vi "Create Channel and Node Pair.vi"(8 "Port ID":string, 9 "Node ID":string, 10 "name":string, 11 "Instance ID":string) -> (3 "Channel to Port Pair":T1)   [LabVIEW 2014, in "GraphViz Mapping Visualizer.lvlib"]
uses:
  GraphViz Mapping Visualizer.lvlib
  Channel to Port Pair.ctl
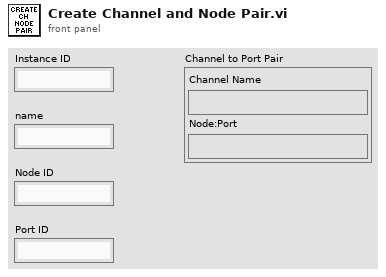
[diagram p1: front panel]
types:
  T1 = typedef "GraphViz Mapping Visualizer.lvlib/Channel to Port Pair.ctl" = cluster{"Channel Name":string, "Node:Port":string}
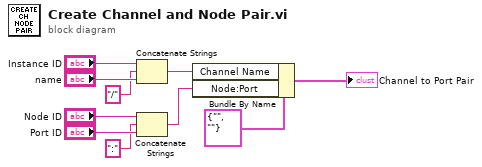
[diagram p0: block diagram]
diagram:
  n1 = Concatenate Strings("Instance ID", "/", "name") -> (w6:string)
  n2 = Concatenate Strings("Node ID", ":" ("string"), "Port ID") -> (w4:string)
  n3 = Bundle By Name(cluster=T1 {"Channel Name"="", "Node:Port"=""} ("Channel to Port Pair"), "Channel Name"=w6, "Node:Port"=w4) -> (→"Channel to Port Pair":T1)
